vi "TurnAngleOperation.vi"(7 "RobotDriveRef in":T1={"RobotDriveDevRef"={"DevStatus"={"status"=FALSE, "code"=0, "source"=""}, "Motors[]"=[], "Square Inputs"=FALSE, "Max Output"=0.0}, "Control Mode"=enum."Percent VBus", "Motor Settings"={"Wheel Radius"=0.0, "Encoder Ticks Per Rev"=0.0, "Gear Ratio"=0.0, "ClimbRev"=0.0}, "Default Control Mode"=enum."Unchanged / Invalid"}, 8 "error in (no error)":errorcluster, 9 "SubSystem Data":T10, 10 "Control Mode":T8, 11 "Command Loop Data":cluster{"Start Time (ms)":u32, "Iterations":i32}) -> (0 "error out":errorcluster, 1 "Left Motor Value":dbl, 2 "RobotDriveRef out":T1={"RobotDriveDevRef"={"DevStatus"={"status"=FALSE, "code"=0, "source"=""}, "Motors[]"=[], "Square Inputs"=FALSE, "Max Output"=0.0}, "Control Mode"=enum."Percent VBus", "Motor Settings"={"Wheel Radius"=0.0, "Encoder Ticks Per Rev"=0.0, "Gear Ratio"=0.0, "ClimbRev"=0.0}, "Default Control Mode"=enum."Unchanged / Invalid"}, 3 "Wait Time":dbl, 4 "Waveform Chart":cluster{"output":dbl, "Angle":dbl, "Yaw":dbl}(graph), 5 "Finished":bool, 6 "Right Motor Value":dbl)   [LabVIEW 2015]
uses:
  Drive Setpoints.ctl
  Drive Operations.ctl
  Advanced Drive VIs/RobotDrive Type Def.ctl
  <vilib>/Rock Robotics/WPI/MotorControl/WPI_MotorControlDeviceRef.ctl
  <vilib>/Rock Robotics/WPI/MotorControl/WPI_MotorControlType.ctl
  <vilib>/Rock Robotics/SystemInterfaces/DIO/FPGA_DIOPWMChannel.ctl
  <vilib>/Rock Robotics/WPI/PWM/WPI_PWMDeadband.ctl
  <vilib>/Rock Robotics/WPI/CAN/Jaguar/SubVIs/WPI_CANJaguar_ControlMode.ctl
  <vilib>/Rock Robotics/WPI/CAN/TalonSRX/WPI_CANTalonSRX_APIControlMode.ctl
  Advanced Drive VIs/Drive Motor Settings.ctl
  NavX/NavX Global.vi
  <vilib>/addons/control/pid/pid.llb/PID (DBL).vi
  <vilib>/Rock Robotics/WPI/Joystick/WPI_JoystickArcadeMapping.vi
  <vilib>/addons/control/pid/NI_PID_pid.lvlib
  NavX/Library/navX Library v2.lvlib
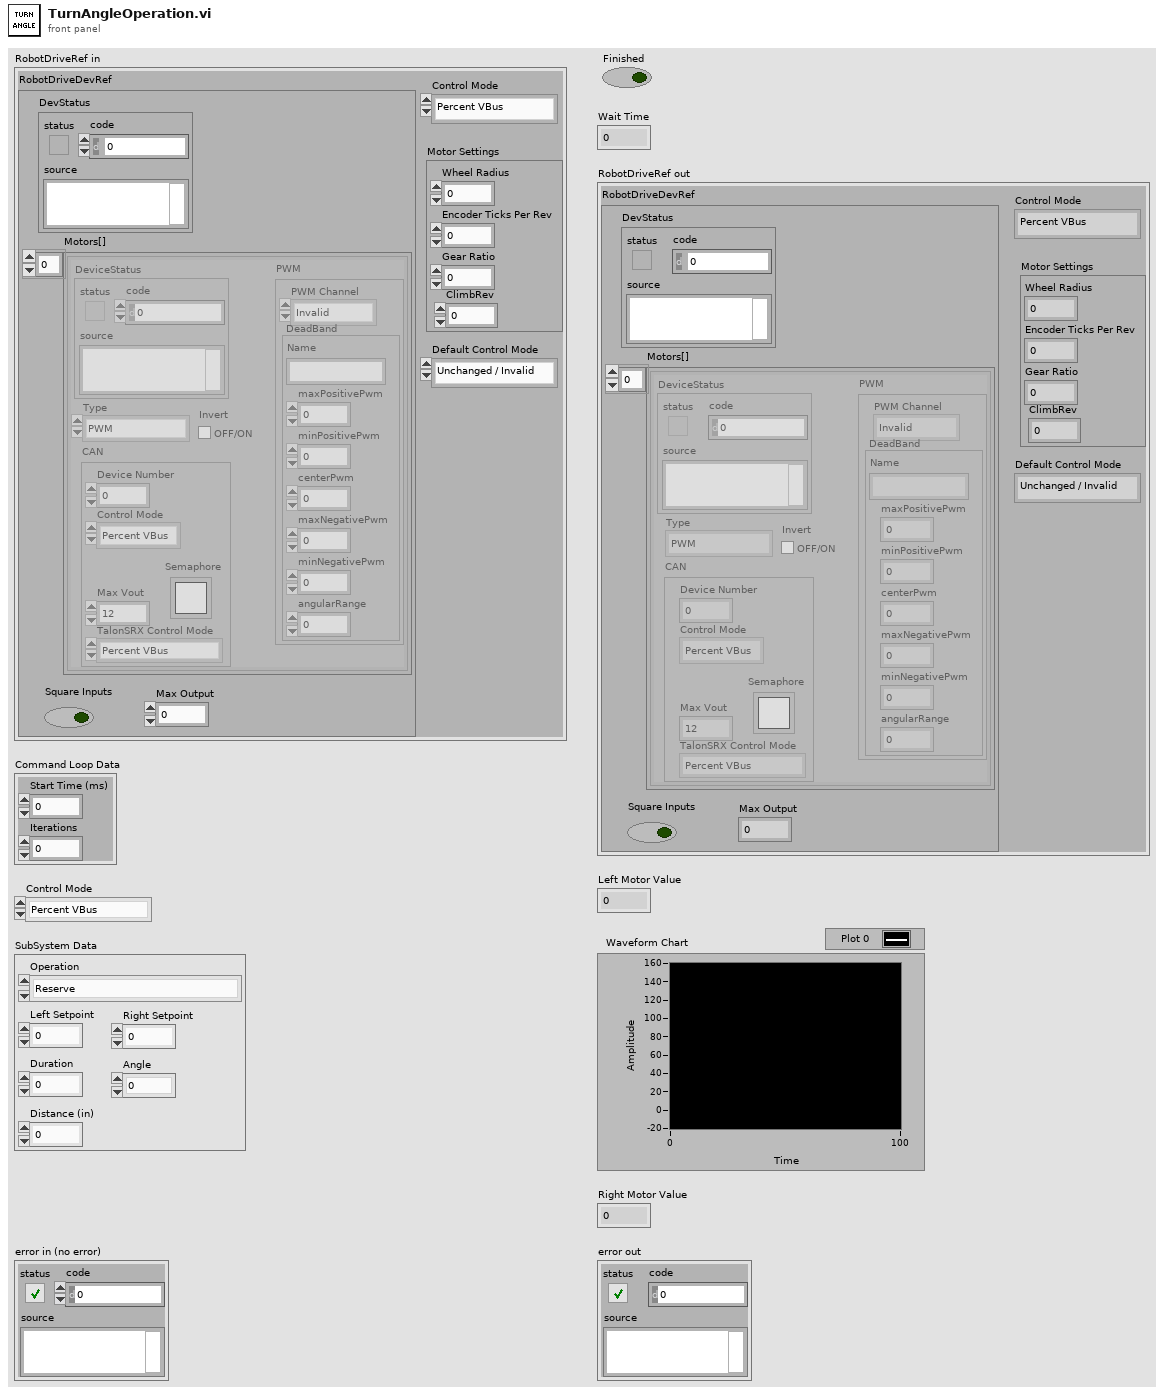
[diagram p1: front panel]
types:
  T1 = typedef "RobotDrive Type Def.ctl" = cluster{"RobotDriveDevRef":cluster{"DevStatus":errorcluster, "Motors[]":T2[], "Square Inputs":bool, "Max Output":dbl}, "Control Mode":T8, "Motor Settings":T9, "Default Control Mode":T8}
  T2 = typedef "WPI_MotorControlDeviceRef.ctl" = cluster{"DeviceStatus":errorcluster, "Type":T3, "PWM":cluster{"PWM Channel":T4, "DeadBand":T5}, "CAN":cluster{"Device Number":u8, "Control Mode":T6, "Semaphore":T7, "Max Vout":dbl, "TalonSRX Control Mode":T8}, "Invert":bool}
  T3 = typedef "WPI_MotorControlType.ctl" = enum16{"PWM", "CAN", "CANTalonSRX"}
  T4 = typedef "FPGA_DIOPWMChannel.ctl" = enum8{"PWM 0", "PWM 1", "PWM 2", "PWM 3", "PWM 4", "PWM 5", "PWM 6", "PWM 7", "PWM 8", "PWM 9", "PWM MXP 0", "PWM MXP 1", "PWM MXP 2", "PWM MXP 3", "PWM MXP 4", "PWM MXP 5", "PWM MXP 6", "PWM MXP 7", "PWM MXP 8", "PWM MXP 9", "Invalid"}
  T5 = typedef "WPI_PWMDeadband.ctl" = cluster{"Name":string, "maxPositivePwm":i32, "minPositivePwm":i32, "centerPwm":i32, "maxNegativePwm":i32, "minNegativePwm":i32, "angularRange":u16}
  T6 = typedef "WPI_CANJaguar_ControlMode.ctl" = enum8{"Percent VBus", "Current", "Speed", "Position", "Voltage"}
  T7 = typedef "Semaphore RefNum" = refnum<k1>
  T8 = typedef "WPI_CANTalonSRX_APIControlMode.ctl" = enum8{"Percent VBus", "Speed", "Position", "Slave", "Unchanged / Invalid", "Voltage Compensation", "Current", "Motion Profile"}
  T9 = typedef "Drive Motor Settings.ctl" = cluster{"Wheel Radius":dbl, "Encoder Ticks Per Rev":dbl, "Gear Ratio":dbl, "ClimbRev":dbl}
  T10 = typedef "Drive Setpoints.ctl" = cluster{"Operation":T11, "Left Setpoint":dbl, "Right Setpoint":dbl, "Duration":dbl, "Angle":dbl, "Distance (in)":dbl}
  T11 = typedef "Drive Operations.ctl" = enum16{"Reserve", "Read Current", "Immediate", "Drive for Time", "Drive for Distance", "Turn Degrees"}
  T12 = cluster{"proportional gain (Kc)":dbl, "integral time (Ti, min)":dbl, "derivative time (Td, min)":dbl}
  T13 = cluster{"Yaw":dbl, "Roll":dbl, "Pitch":dbl, "Heading":dbl, "Fused Heading":dbl}
  T14 = typedef "navX Library v2.lvlib/Z900_navX_DeviceTypeDef.ctl" = cluster{"Interface":cluster{"Protocol":T15, "Update Rate (4Hz-60Hz)":u8, "navX Open TypeDef":variant}, "Notify Packet":refnum<notifier>, "Loop VI Refnum":refnum<vi>, "Ready to Close Occurrence Refnum":refnum<k4>}
  T15 = typedef "navX Library v2.lvlib/Z900_navX_ProtocolTypeDef.ctl" = enum16{"SERIAL", "I2C", "SPI"}
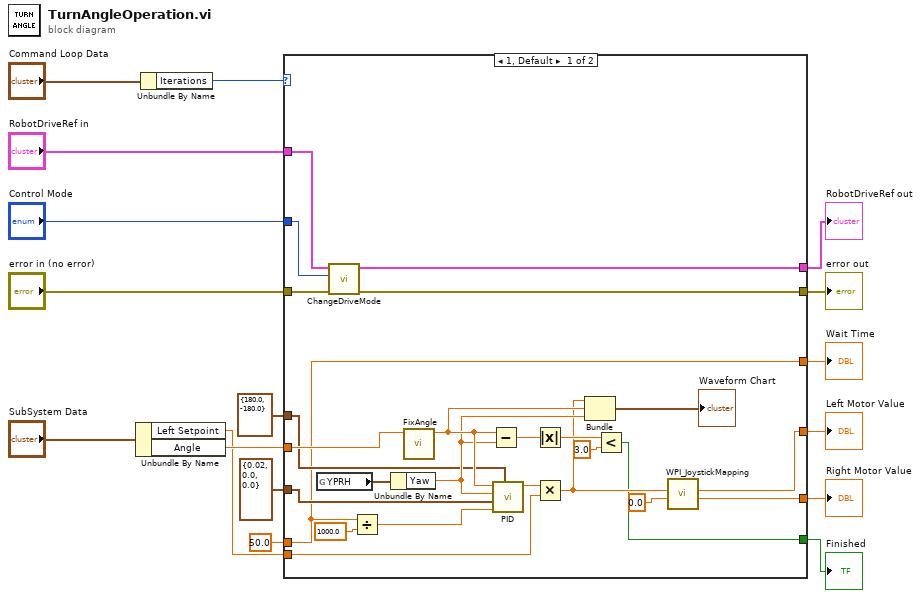
[diagram p0: block diagram]
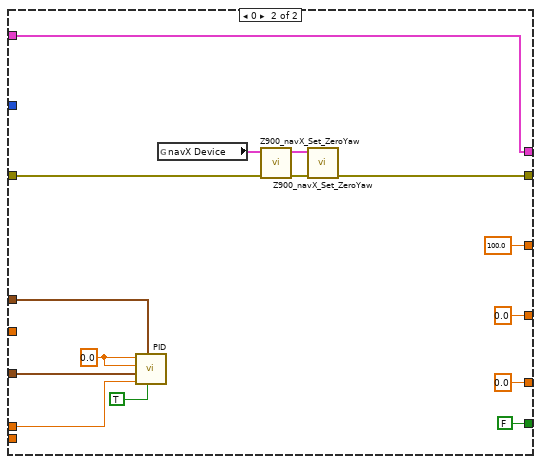
[diagram p2: hidden frame]
diagram:
  n1 = Unbundle By Name("SubSystem Data") -> ("Left Setpoint"=w16:dbl, "Angle"=w17:dbl)
  n2 = Unbundle By Name("Command Loop Data") -> ("Iterations"=w9:i32)
  n3 = case shown="1, Default" w9 {
    tunnel: [w42 0.0 ("Left Motor Value")] -> w3
    tunnel: [w41 0.0 ("Right Motor Value")] -> w4
    tunnel: "RobotDriveRef in" -> [w38 w55]
    tunnel: "Control Mode" -> [w37 _]
    tunnel: [w36 w55] -> w7
    tunnel: w17 -> [w31 _]
    tunnel: w16 -> [w21 _]
    tunnel: cluster{"output high":dbl, "output low":dbl} {"output high"=180.0, "output low"=-180.0} ("output range") -> [w26 w50]
    tunnel: 50.0 -> [w19 w53]
    tunnel: T12 {"proportional gain (Kc)"=0.02, "integral time (Ti, min)"=0.0, "derivative time (Td, min)"=0.0} ("PID gains") -> [w25 w52]
    tunnel: "error in (no error)" -> [w24 w44]
    tunnel: [w23 w43] -> w13
    tunnel: [w22 FALSE] -> w14
    tunnel: [w19 100.0] -> w2
    frame 1, Default {
      n4 = global read "NavX Global.vi" "YPRH"() -> (w39:T13)
      n5 = call "ChangeDriveMode.vi"("error in (no error)"=w24, "Control Mode"=w37, "RobotDriveRef"=w38) -> ("error out"=w23:errorcluster, "RobotDriveRef Out"=w36:T1)  [unwired: 7 in]
      n6 = Divide(x=w19, y=1000.0) -> (x/y=w18:dbl)
      n7 = Unbundle By Name(w39) -> ("Yaw"=w29:dbl)
      n8 = call "FixAngle.vi"("Angle To Turn in"=w31) -> ("Angle To Turn out"=w30:dbl)  [unwired: 10 in]
      n9 = Subtract(x=w30, y=w29) -> (x-y=w34:dbl)
      n10 = call-poly <vilib>:"PID.vi"("output range"=w26, "dt (s)"=w18, "PID gains"=w25, "process variable"=w29, "setpoint"=w30) -> ("output"=w27:dbl)  [unwired: 5 in, 1 out]
      n11 = Absolute Value(x=w34) -> (abs(x)=w33:dbl)
      n12 = Multiply(x=w27, y=w21) -> (x*y=w28:dbl)
      n13 = Bundle(w28, "Angle To Turn out"=w30, "Yaw"=w29) -> (→"Waveform Chart":cluster{dbl, "Angle To Turn out":dbl, "Yaw":dbl})  [unwired: 1 in]
      n14 = Less?(x=w33, y=3.0) -> (x < y?=w22:bool)
      n15 = call-poly <vilib>:"WPI_JoystickMapping.vi"("Y axis value"=0.0, "X axis value"=w28) -> ("Right Motor Value"=w41:dbl, "Left Motor Value"=w42:dbl)  [unwired: 8 in]
    }
    frame 0 {
      w51 = 0.0 ("process variable")
      n16 = call-poly <vilib>:"PID.vi"("reinitialize? (F)"=TRUE, "output range"=w50, "dt (s)"=w53, "PID gains"=w52, "process variable"=w51, "setpoint"=w51) -> ()  [unwired: 4 in, 2 out]
      n17 = global read "NavX Global.vi" "navX Device"() -> (w47:T14)
      n18 = call "Z900_navX_Set_ZeroYaw.vi"("error in (no error)"=w44, "navX Device"=w47) -> ("error out"=w45:errorcluster, "navX Device"=w46:T14)  [unwired: 8 in]
      n19 = call "Z900_navX_Set_ZeroYaw.vi"("error in (no error)"=w45, "navX Device"=w46) -> ("error out"=w43:errorcluster)  [unwired: 8 in, 1 out]
    }
  }
  "Finished" <- w14
  "error out" <- w13
  "Wait Time" <- w2
  "RobotDriveRef out" <- w7
  "Right Motor Value" <- w4
  "Left Motor Value" <- w3
